vi "Signal Average_y.vi"(11 "Filtered Correction":dbl=0.1 format="%#_13g") -> (3 "Average Signal":dbl)   [LabVIEW 2019]
panel:
  in  "iterations":i32=100
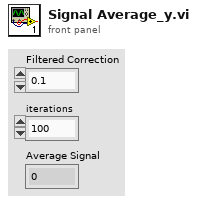
[diagram p1: front panel]
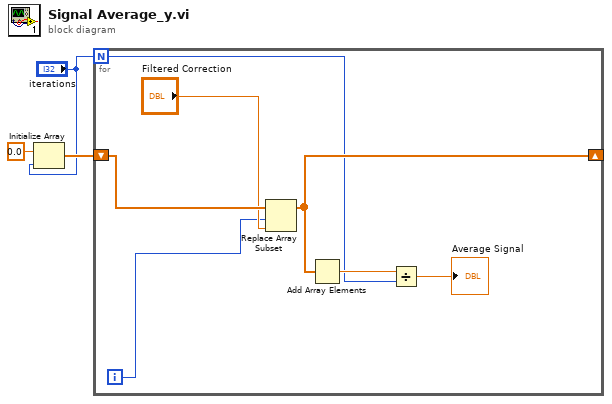
[diagram p0: block diagram]
diagram:
  n1 = Initialize Array(0.0 ("element"), "iterations") -> (w2:dbl[])
  n2 = for {
    N: "iterations" -> [w4]
    shift-right: [w8] -> _
    shift-left: w2 -> [w10]
    i -> [w5]
    n3 = Replace Array Subset(array=w10, new element="Filtered Correction", index=w5) -> (w8:dbl[])
    n4 = Add Array Elements(numeric array=w8) -> (sum=w7:dbl)
    n5 = Divide(x=w7, y=w4) -> (x/y=→"Average Signal":dbl)
  }
